vi "Hardware Configuration Global.vi"() -> ()   [LabVIEW 2013]
panel:
  in  "Blocking Signal Generator":refnum<k15>="PXI1Slot3"
  in  "Wanted Signal Generator":refnum<k15>="PXI1Slot2"
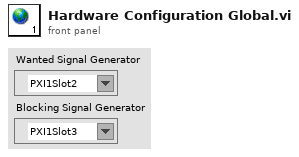
[diagram p1: front panel]
diagram:
